vi "text_colors.vi"() -> ()   [LabVIEW 2019]
panel:
  in  "Text.Colors:BG Color":u32(colorbox)
  out "String 2":string
  in  "Disabled":T1(ring)
  in  "Boolean":bool
  out "concatenated string":string
  in  "stop":bool
  in  "String":string
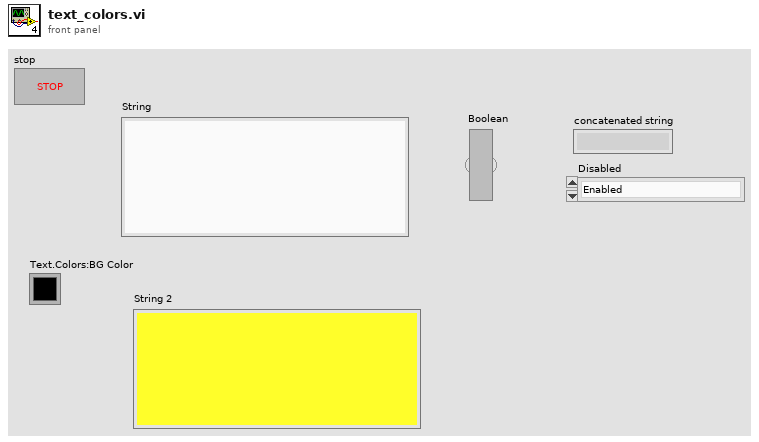
[diagram p1: front panel]
types:
  T1 = enum8{"Enabled", "Disabled", "Disabled and Grayed Out"}
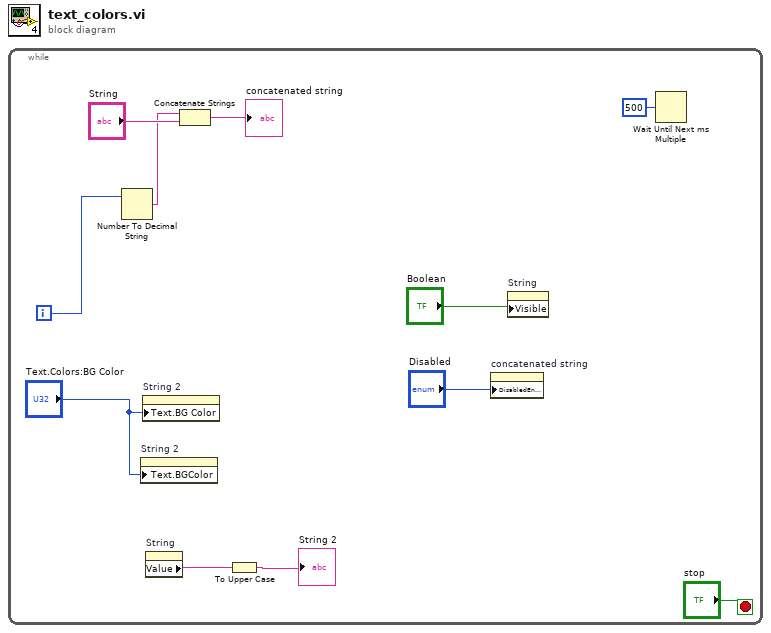
[diagram p0: block diagram]
diagram:
  n1 = while {
    i -> [w11]
    stop <- "stop" stop-if-true
    n2 = Number To Decimal String(number=w11) -> (decimal integer string=w8:string)  [unwired: 1 in]
    n3 = property on="String 2" class="Str"("Text.BGColor"="Text.Colors:BG Color") -> ()  [unwired: 2 in, 2 out]
    n4 = property on="String 2" class="Str"("Text.BG Color"="Text.Colors:BG Color") -> ()  [unwired: 2 in, 2 out]
    n5 = property on="String" class="Str"() -> ("Value"=w2:string)  [unwired: 2 in, 2 out]
    n6 = Concatenate Strings(w8, "String") -> (→"concatenated string":string)
    n7 = To Upper Case(1:w2) -> (0:→"String 2":string)
    n8 = property on="concatenated string" class="Str"("DisabledEnum"="Disabled") -> ()  [unwired: 2 in, 2 out]
    n9 = property on="String" class="Str"("Visible"="Boolean") -> ()  [unwired: 2 in, 2 out]
    n10 = Wait Until Next ms Multiple(millisecond multiple=u32 500) -> ()  [unwired: 1 out]
  }
